vi "p1.vi"() -> ()   [LabVIEW 2023, in "d1.lvlib"]
uses:
  d1.lvlib
  <vilib>/regexp/Match Regular Expression.xnode
  AOC/AOC.lvlib
panel:
  in  "Input":string="sixrrmlkptmc18zhvninek\njcb82eightwond\ntwofourthree778nineeight\nsqpxs1cgcrmctlgqvzxbcjzgr\nnqkjxbmbpkz9eight8\none6fourfiveqndtrvgkkgthppnine\nzbrbdpbfcfxcqq5oneninejfgqpkfn\nhvlstzgvmjfivefourqjqtxdjmbxfour4four2\n13dzbmbtl6\nfourone2pmlxzzbmnfxg2\n3fourrbvvlrsrbb2858\nvlz4six89\n75threeb\nfourp783fiveseventhree\n2gxvcbsmn6\n896\ndnblxtxxpstlsix56\n4fivecl185\nonefk8sdljtfv37zsxsxrv7qvrpnmd\nfourdvhzp7foursix\nseventwonineseven27jbrqpxfx8\n1threenine241gnrdfqn5\nsixnrsqdgmkvs7sevenkgjgtglmdq9dkdzsdqmq2nptbxnxghm\nllbkdcpxkg1tnmnmrbskpdb\nzb7nvjz1eighttwo6nine\n5threeeightwor\ntgjmdbr4sixone5\n4twoseven7tjmklbl\nlt2vqg..."
  in  "Example":string="1abc2\npqr3stu8vwx\na1b2c3d4e5f\ntreb7uchet"
  in  "Example?":bool
  out "Answer":i64=55607
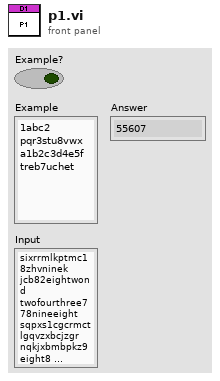
[diagram p1: front panel]
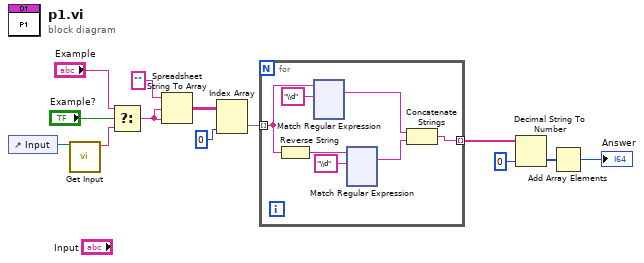
[diagram p0: block diagram]
diagram:
  n1 = control-ref of="Input"() -> (w1:refnum<vi>)
  n2 = call "Get Input.vi"("Input ref"=w1) -> ("Input"=w12:string)  [unwired: 10 in]
  n3 = Select(t="Example", s="Example?", f=w12) -> (s? t:f=w10:string)
  n4 = Spreadsheet String To Array(format string="", spreadsheet string=w10, array type (2D Dbl)=w10) -> (array=w4:string[][])  [unwired: 1 in]
  n5 = Index Array(array=w4, index (col)=0 ("disabled index (col)")) -> (element=w2:string[])  [unwired: 1 in]
  n6 = for {
    tunnel: w2 -> [w19] mode=indexing
    tunnel: [w14] -> w9 mode=indexing
    n7 = Reverse String(1:w19) -> (0:w17:string)
    n8 = xnode "Match Regular Expression"("input string"=w19, "regular expression"="\\d") -> ("whole match"=w15:string)  [unwired: 4 in, 4 out]
    n9 = xnode "Match Regular Expression"("input string"=w17, "regular expression"="\\d") -> ("whole match"=w16:string)  [unwired: 4 in, 4 out]
    n10 = Concatenate Strings(w15, w16) -> (w14:string)
  }
  n11 = Decimal String To Number(string=w9, default (0L)=i64 0 ("default (0 I32)")) -> (number=w7:i64[])  [unwired: 1 in, 1 out]
  n12 = Add Array Elements(numeric array=w7) -> (sum=→"Answer":i64)
